vi "test2.vi"() -> ()   [LabVIEW 2023]
panel:
  in  "Filename":path=path "test.lvm"
  out "Waveform Graph":dynamicdata(graph)
  in  "Amplitude (V)":dbl(knob) scale=0.0..5.0
  in  "Frequency (Hz)":dbl(knob) scale=0.0..20.0
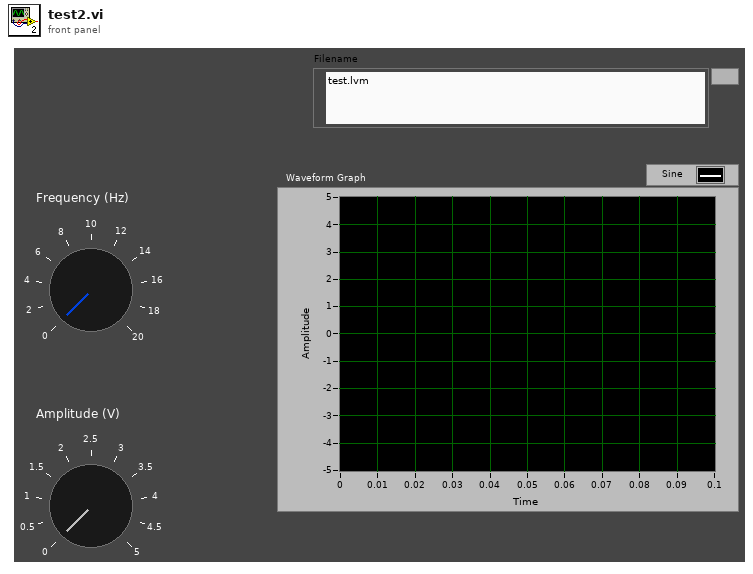
[diagram p1: front panel]
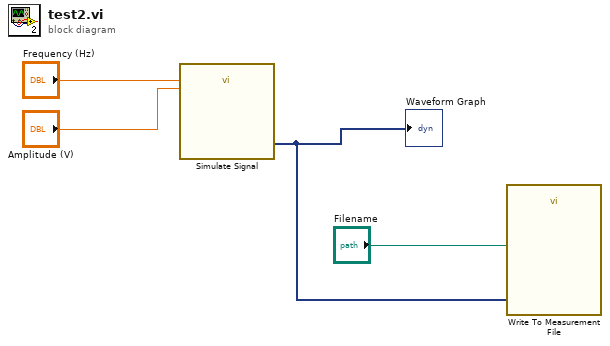
[diagram p0: block diagram]
diagram:
  n1 = call "Simulate Signal"("Frequency"="Frequency (Hz)", "Amplitude"="Amplitude (V)") -> ("Sine"=w2:dynamicdata)  [unwired: 12 in, 1 out]
  "Waveform Graph" <- w2
  n2 = call "Write To Measurement File"("Signals"=w2, "Filename"="Filename") -> ()  [unwired: 15 in, 3 out]
